vi "GetAttribute.vi"(0 "reference in":refnum<class "G#BaseClass1.lvclass">, 5 "error in (no error)":errorcluster) -> (14 "reference out":refnum<class "G#BaseClass1.lvclass">, 16 "Numeric":dbl, 17 "Array":dbl[](array[numeric]), 19 "error out":errorcluster)   [LabVIEW 2020, in "G#BaseClass1.lvclass"]
uses:
  G#BaseClass1.lvclass
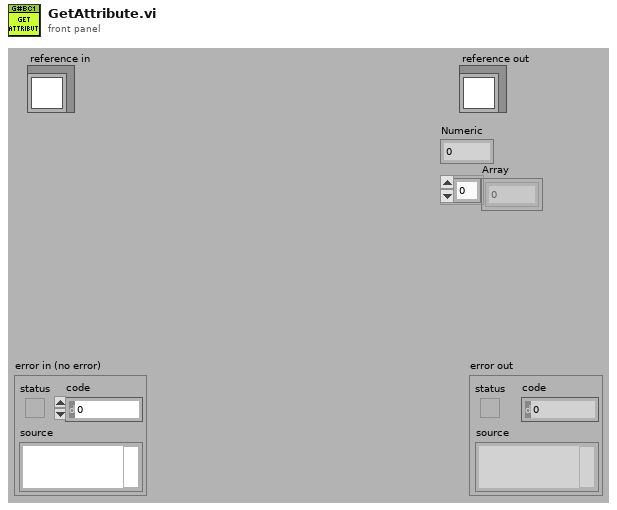
[diagram p1: front panel]
types:
  T1 = typedef "G#BaseClass1.lvclass/ObjectAttributes.ctl" = cluster{"Numeric":dbl, "Array":dbl[]}
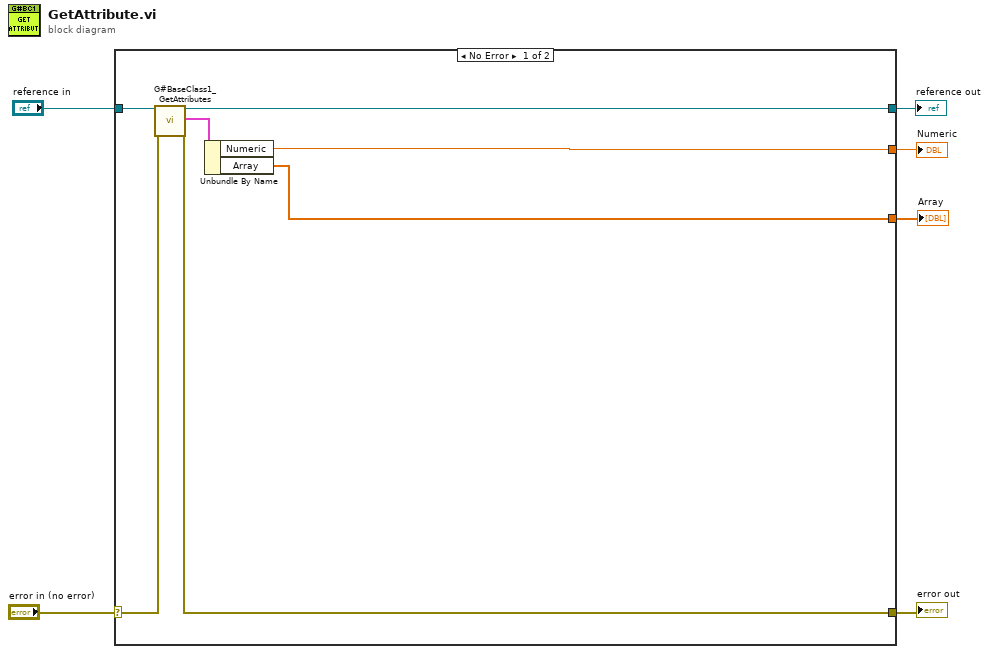
[diagram p0: block diagram]
diagram:
  n1 = case shown="No Error" "error in (no error)" {
    selector: "error in (no error)" -> [w13 w15]
    tunnel: [w11 w15] -> w5
    tunnel: [w9 w14] -> w3
    tunnel: "reference in" -> [w10 w14]
    tunnel: [w8 _] -> w2
    tunnel: [w7 _] -> w1
    frame No Error {
      n2 = call "G#BaseClass1_GetAttributes.vi"("reference in"=w10, "error in (no error)"=w13) -> ("reference out"=w9:refnum<class "G#BaseClass1.lvclass">, "attributes"=w12:T1, "error out"=w11:errorcluster)  [unwired: 14 in, 1 out]
      n3 = Unbundle By Name(w12) -> ("Numeric"=w8:dbl, "Array"=w7:dbl[])
    }
    frame Error {
    }
  }
  "error out" <- w5
  "reference out" <- w3
  "Numeric" <- w2
  "Array" <- w1
